vi "IncrementBlueSerializableVersion.vi"(8 "error in (no error)":errorcluster, 9 "Version Bump 2":T1, 10 "Version Bump 1":T1, 11 "LabVIEW Object":refnum<class>) -> (0 "error out":errorcluster, 3 "New BlueSerializableVersion":u16)   [LabVIEW 2019, in "IncrementMutationHistory.lvlib"]
uses:
  IncrementMutationHistory.lvlib
  <vilib>/Utility/EditLVLibs/LibVersion.ctl
  <resource>/Framework/Providers/BlueSerializationProviderShared/UserCommentToVersion.vi
  <vilib>/Utility/error.llb/Error Cluster From Error Code.vi
  <vilib>/ErrorRing/Error Ring.xnode
  <resource>/Framework/Providers/BlueSerializationProviderShared/BlueSerializationProviderShared.lvlib
  VILIB_NONUI/VILIB_NONUI.lvlib
  <vilib>/Utility/EditLVLibs/Edit LVLibs.lvlib
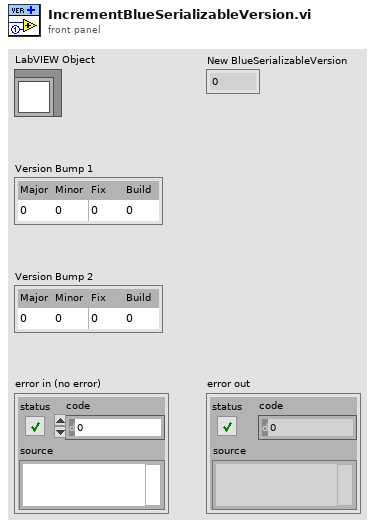
[diagram p1: front panel]
types:
  T1 = typedef "Edit LVLibs.lvlib/LibVersion.ctl" = cluster{"Major":u16, "Minor":u16, "Fix":u16, "Build":u16}
  T2 = typedef "Edit LVLibs.lvlib/Mutation History.ctl" = T3[]
  T3 = typedef "Edit LVLibs.lvlib/Mutation Record.ctl" = cluster{"Library Version":T1, "Old Name Index":u8, "Class Default Data":variant, "Cluster Order Map":u32[], "Parent Name":string, "Parent Path":path, "LabVIEW Version":u32, "User Comments":string, "Mutation Flags":u8, "Parent Old Name Index":u8, "Parent Levels Added":u16, "Parent Levels Removed":u16}
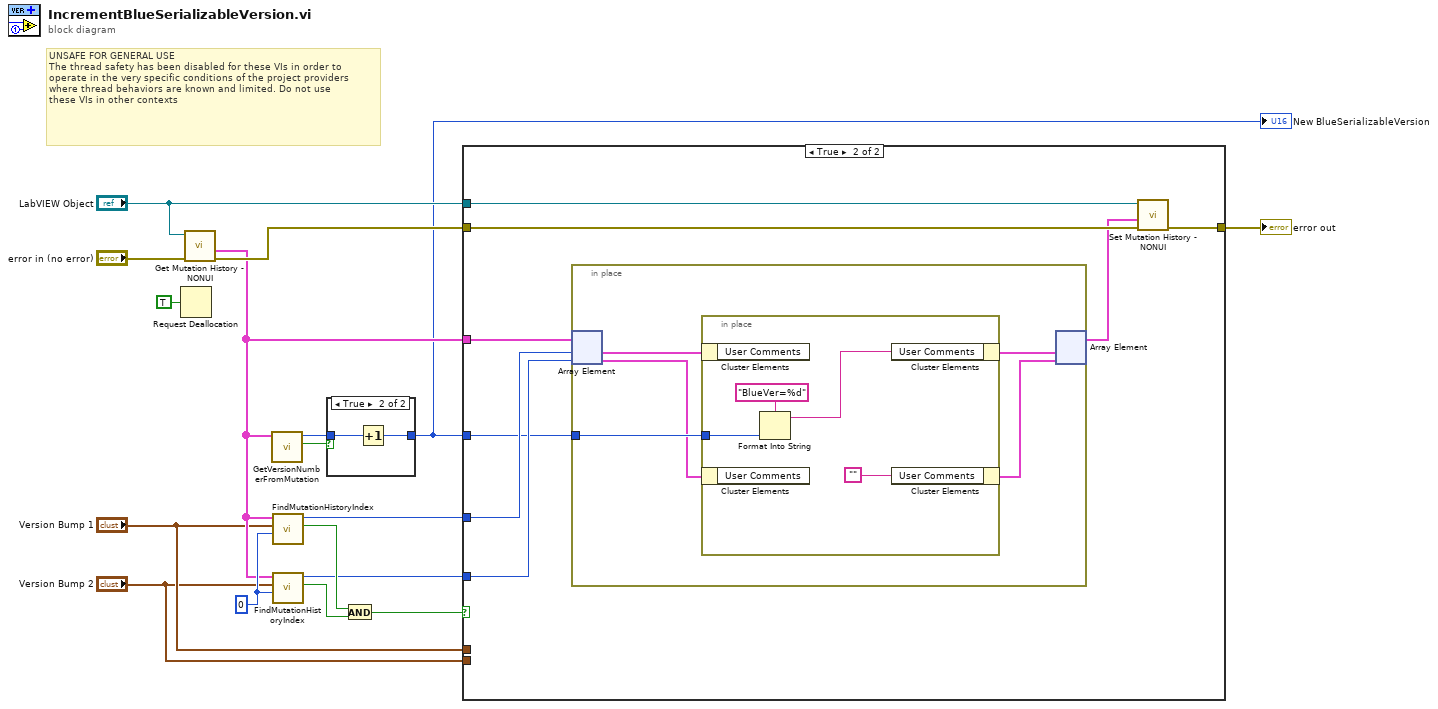
[diagram p0: block diagram]
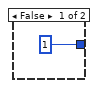
[diagram p2: hidden frame]
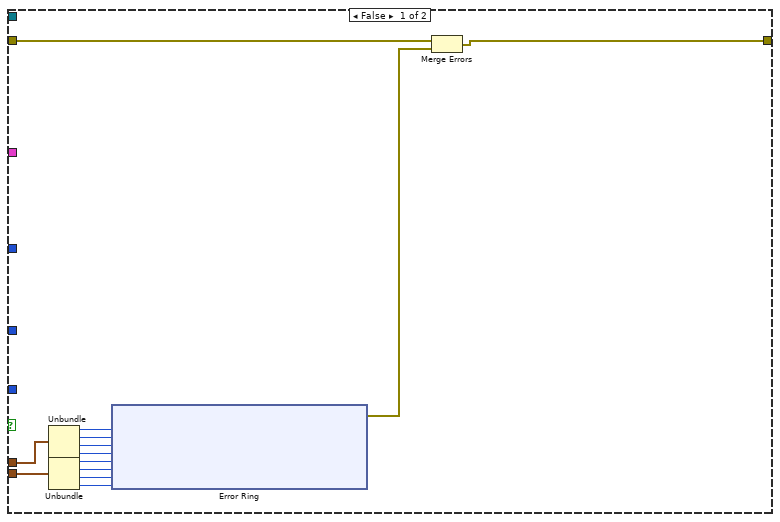
[diagram p3: hidden frame]
diagram:
  w10 = u8 0 ("Old Name Index")
  # "UNSAFE FOR GENERAL USE\nThe thread safety has been disabled for these VIs in order to\noperate in the very specific conditions of the project providers\nwhere thread behaviors are known and limited. Do not use\nthese VIs in other contexts"
  n1 = Request Deallocation(TRUE ("flag")) -> ()
  n2 = call "Get Mutation History - NONUI.vi"("error in"="error in (no error)", "Input object"="LabVIEW Object") -> ("error out"=w15:errorcluster, "Mutation History"=w5:T2)  [unwired: 6 in]
  n3 = call <resource>:"GetVersionNumberFromMutation.vi"("Mutation History"=w5) -> ("BlueSerializableVersion found?"=w11:bool, "BlueSerializableVersion"=w12:u16)  [unwired: 9 in]
  n4 = call <resource>:"FindMutationHistoryIndex.vi"("Old Name Index"=w10, "Library Version"="Version Bump 1", "Mutation History"=w5) -> ("Found?"=w8:bool, "Index"=w7:i32)  [unwired: 7 in]
  n5 = call <resource>:"FindMutationHistoryIndex.vi"("Old Name Index"=w10, "Library Version"="Version Bump 2", "Mutation History"=w5) -> ("Found?"=w9:bool, "Index"=w6:i32)  [unwired: 7 in]
  n6 = case shown="True" w11 {
    tunnel: w12 -> [_ w20]
    tunnel: [u16 1 w19] -> w4
    frame False {
    }
    frame True {
      n7 = Increment(x=w20) -> (x+1=w19:u16)
    }
  }
  "New BlueSerializableVersion" <- w4
  n8 = And(x=w8, y=w9) -> (x .and. y?=w3:bool)
  n9 = case shown="True" w3 {
    tunnel: "LabVIEW Object" -> [_ w55]
    tunnel: w15 -> [w23 w54]
    tunnel: [w21 w53] -> w14
    tunnel: w7 -> [_ w52]
    tunnel: w6 -> [_ w51]
    tunnel: w5 -> [_ w50]
    tunnel: w4 -> [_ w49]
    tunnel: "Version Bump 1" -> [w33 _]
    tunnel: "Version Bump 2" -> [w32 _]
    frame False {
      n10 = Unbundle(w33) -> ("Major"=w30:u16, "Minor"=w31:u16, "Fix"=w29:u16, "Build"=w28:u16)
      n11 = Unbundle(w32) -> ("Major"=w27:u16, "Minor"=w26:u16, "Fix"=w25:u16, "Build"=w24:u16)
      n12 = xnode "Error Ring"("parameter 0"=w30, "parameter 1"=w31, "parameter 2"=w29, "parameter 3"=w28, "parameter 4"=w27, "parameter 5"=w26, "parameter 6"=w25, "parameter 7"=w24) -> ("error out"=w22:errorcluster)
      n13 = Merge Errors(w23, w22) -> (w21:errorcluster)
    }
    frame True {
      n14 = in-place {
        in-place-border: w49 -> [w60]
        n15 = in-place-array #1(w50, w52, w51) -> (w59:T3, w57:T3)
        n16 = in-place {
          in-place-border: w60 -> [w63]
          n17 = in-place-cluster #2(w59) -> ()  [unwired: 1 out]
          n18 = in-place-cluster #3(w57) -> ()  [unwired: 1 out]
          n19 = Format Into String(format string="BlueVer=%d" ("regular expression"), w63) -> (resulting string=w62:string)  [unwired: 2 in, 1 out]
          n20 = in-place-cluster #2("User Comments"=w62) -> (w58:T3)
          n21 = in-place-cluster #3("User Comments"="") -> (w56:T3)
        }
        n22 = in-place-array #1(w58, w56) -> (w48:T2)  [unwired: 2 out]
      }
      n23 = call "Set Mutation History - NONUI.vi"("error in"=w54, "Mutation History"=w48, "Input object"=w55) -> ("error out"=w53:errorcluster)  [unwired: 8 in]
    }
  }
  "error out" <- w14
